vi "XNET IP Stack Get Info.vi"(0 "stack in":refnum<k21>, 11 "error in":errorcluster) -> (4 "stack out":refnum<k21>, 6 "stack info":T1[](array[typedef]) {"operational status" items=["Down", "Up"]; "gateway address list"."address family" items=["IPv4"=2, "IPv6"=10]; "IP address list"."address family" items=["IPv4"=2, "IPv6"=10]}, 15 "error out":errorcluster)   [LabVIEW 2018]
doc: "Gets runtime information for an XNET IP Stack."
uses:
  XNET IP Stack Virtual Interface Info.ctl
  XNET IP Stack Operational Status.ctl
  XNET IP Stack IP Address Info.ctl
  XNET IP Stack Address Family.ctl
  XNET IP Stack Gateway Address Info.ctl
  nixlvapi.dll
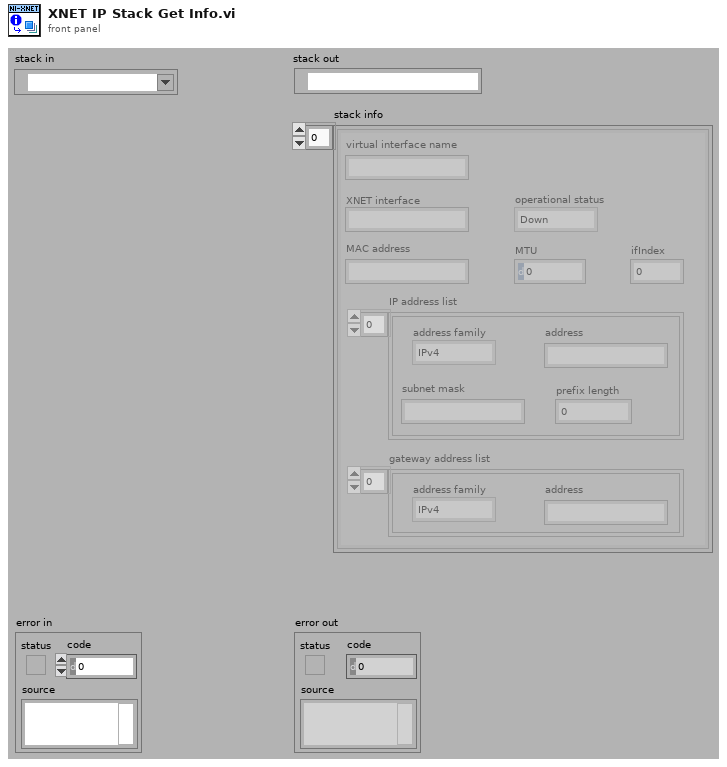
[diagram p1: front panel]
types:
  T1 = typedef "XNET IP Stack Virtual Interface Info.ctl" = cluster{"virtual interface name":string, "XNET interface":string, "operational status":T2, "MAC address":string, "MTU":u32, "ifIndex":u32, "IP address list":T3[], "gateway address list":T5[]}
  T2 = typedef "XNET IP Stack Operational Status.ctl" = u32
  T3 = typedef "XNET IP Stack IP Address Info.ctl" = cluster{"address family":T4, "address":string, "prefix length":u32, "subnet mask":string}
  T4 = typedef "XNET IP Stack Address Family.ctl" = u32
  T5 = typedef "XNET IP Stack Gateway Address Info.ctl" = cluster{"address family":T4, "address":string}
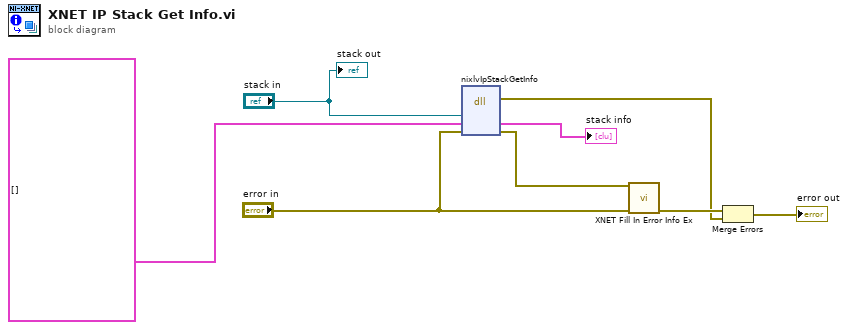
[diagram p0: block diagram]
diagram:
  n1 = dll-call lib="nixlvapi.*" fn="nixlvIpStackGetInfo" label="Call Library"("reference"="stack in", "stackInfo"=T1[] [] ("stack info"), "errorInOut"="error in") -> (error out=w6:errorcluster, "stackInfo"=→"stack info":T1[], "errorInOut"=w8:errorcluster)  [unwired: 3 in, 3 out]
  n2 = call "XNET Fill In Error Info Ex.vi"("error xnet"=w8, "error in"="error in") -> ("error out"=w7:errorcluster)  [unwired: 13 in]
  n3 = Merge Errors(w7, w6) -> (→"error out":errorcluster)
  "stack out" <- "stack in"
